vi "video.update_set_name.vi"(8 "error in":errorcluster, 11 "VideoUpdateStaging in":refnum<class "VideoUpdateStaging.lvclass">) -> (0 "error out":errorcluster, 3 "VideoUpdateStaging out":refnum<class "VideoUpdateStaging.lvclass">)   [LabVIEW 2020, in "VideoUpdateStaging.lvclass"]
doc: "Stages a new name for the video being updated."
uses:
  VideoUpdateStaging.lvclass
  VideoUpdateStaging.lvclass/VideoUpdateStaging.ctl
  client.lvlib
panel:
  in  "name":string
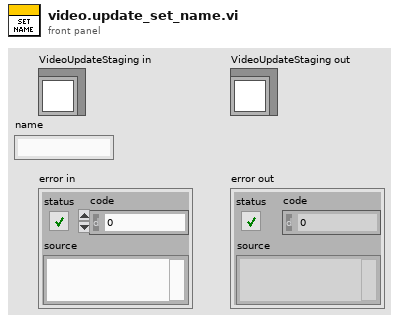
[diagram p1: front panel]
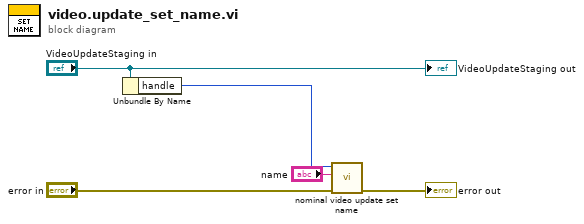
[diagram p0: block diagram]
diagram:
  n1 = Unbundle By Name("VideoUpdateStaging in") -> ("handle"=w3:i32)
  n2 = call "nominal video update set name.vi"("error in (no error)"="error in", "name"="name", "staging"=w3) -> ("error out"=→"error out":errorcluster)  [unwired: 7 in, 1 out]
  "VideoUpdateStaging out" <- "VideoUpdateStaging in"
